vi "DIAdem Request Script.vi"(6 "generator settings":T1={"Wait? (t)"=TRUE, "ClientPrint? (f)"=FALSE, "Client (\"\")"="", "joinPDF"=FALSE, "Sort Method"=enum."Template", "Export Row (-1=all)"=-1, "Preview"=FALSE, "Estimate Time"=FALSE, "username"="", "jobid"=""}, 7 "RunID":string, 8 "error in (no error)":errorcluster, 9 "Queue Entry":enum16{"Front", "Back"}(ring)=enum."Back", 10 "Script Parameters":T2, 11 "TDM File to Load":path) -> (0 "error out":errorcluster, 2 "Timed Out?":bool, 3 "Result":string)   [LabVIEW 2011]
uses:
  Datasheet/CGI Script Parameters.ctl
  Datasheet/Datasheet Generator Settings.ctl
  DIAdem Daemon Queue.ctl
  DIAdem Daemon Script Type.ctl
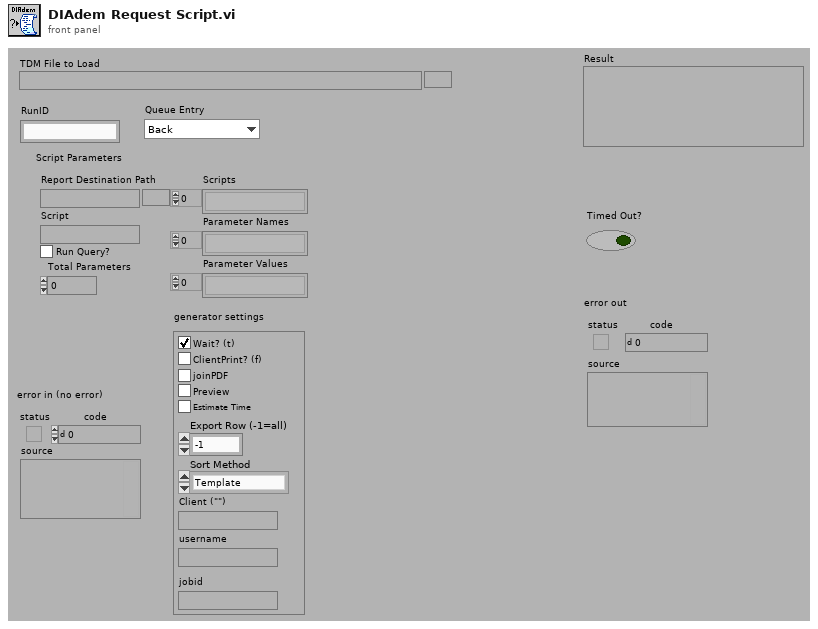
[diagram p1: front panel]
types:
  T1 = typedef "DATASHEET Generator Settings.ctl" = cluster{"Wait? (t)":bool, "ClientPrint? (f)":bool, "Client (\"\")":string, "joinPDF":bool, "Sort Method":enum16{"Item", "Template", "No Sort"}, "Export Row (-1=all)":i32, "Preview":bool, "Estimate Time":bool, "username":string, "jobid":string}
  T2 = typedef "cgi Script parameters.ctl" = cluster{"Report Destination Path":path, "Script":string, "Total Parameters":dbl, "Parameter Names":string[], "Parameter Values":string[], "Scripts":string[], "Run Query?":bool}
  T3 = typedef "DIAdem Daemon Script Type.ctl" = enum16{"Report", "Query", "Script", "Datasheet", "Append", "Restart", "Stop"}
  T4 = typedef "DIAdem Daemon Queue.ctl" = cluster{"Report Template TDM":path, "Report Processor VBS":path, "Report Path PDF":path, "Report Script Params":string, "Username":string, "Script Type":T3, "Report Query Params":string, "Client Machine":string, "Print on Client?":bool, "Response Queue Name":string, "Script Variables":string[], "Start Request Time":timestamp, "Wait?":bool}
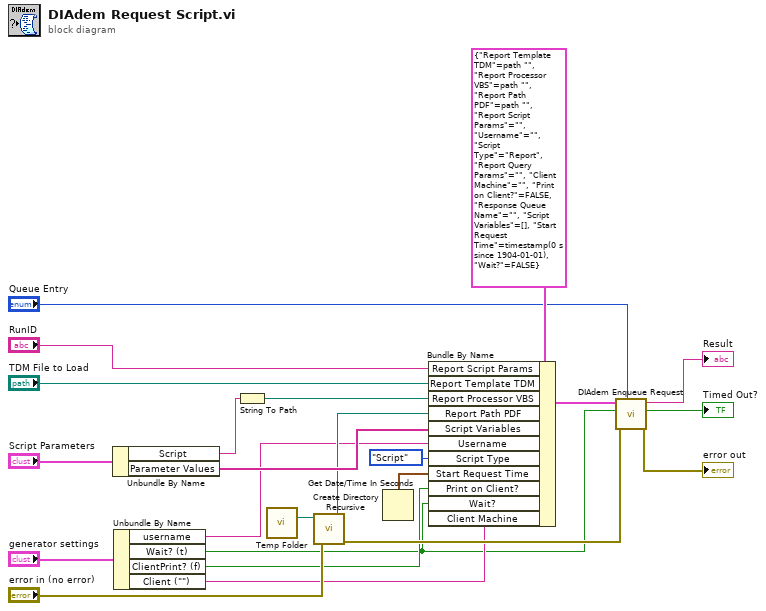
[diagram p0: block diagram]
diagram:
  n1 = Unbundle By Name("Script Parameters") -> ("Script"=w17:string, "Parameter Values"=w18:string[])
  n2 = Unbundle By Name("generator settings") -> ("username"=w4:string, "Wait? (t)"=w1:bool, "ClientPrint? (f)"=w5:bool, "Client (\"\")"=w3:string)
  n3 = String To Path(string=w17) -> (path=w20:path)
  n4 = call "Temp Folder.vi"() -> ("Temp Folder"=w8:path)  [unwired: 3 in]
  n5 = call <vilib>:"Create Directory Recursive.vi"("error in (no error)"="error in (no error)", "directory"=w8) -> ("error out"=w6:errorcluster, "directory copy"=w7:path)  [unwired: 1 in, 3 out]
  n6 = Get Date/Time In Seconds() -> (seconds since 1Jan1904=w10:timestamp)
  n7 = Bundle By Name(cluster=T4 {"Report Template TDM"=path "", "Report Processor VBS"=path "", "Report Path PDF"=path "", "Report Script Params"="", "Username"="", "Script Type"=enum."Report", "Report Query Params"="", "Client Machine"="", "Print on Client?"=FALSE, "Response Queue Name"="", "Script Variables"=[], "Start Request Time"=timestamp(0 s since 1904-01-01), "Wait?"=FALSE} ("DD_Report"), "Report Script Params"="RunID", "Report Template TDM"="TDM File to Load", "Report Processor VBS"=w20, "Report Path PDF"=w7, "Script Variables"=w18, "Username"=w4, "Script Type"=DIAdem_Daemon_Script_Type."Script", "Start Request Time"=w10, "Print on Client?"=w5, "Wait?"=w1, "Client Machine"=w3) -> (w13:T4)
  n8 = call "DIAdem Enqueue Request.vi"("Queue Entry"="Queue Entry", "error in (no error)"=w6, "Wait for Completion? (f)"=w1, "DD_Report"=w13) -> ("error out"=→"error out":errorcluster, "timed out?"=→"Timed Out?":bool, "Results"=→"Result":string)  [unwired: 1 in, 4 out]
